vi "Remove Annotation.vi"(0 "FSM.Graph In":refnum<class "FSM.Graph.lvclass">, 7 "Name":string) -> (4 "FSM.Graph Out":refnum<class "FSM.Graph.lvclass">)   [LabVIEW 2020, in "FSM.Graph.lvclass"]
uses:
  FSM.Graph.lvclass
  FSM.Graph.lvclass/FSM.Graph.ctl
  FSM.Edge/FSM.Edge.lvclass
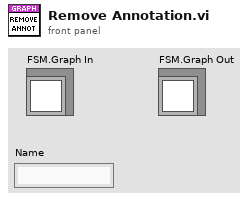
[diagram p1: front panel]
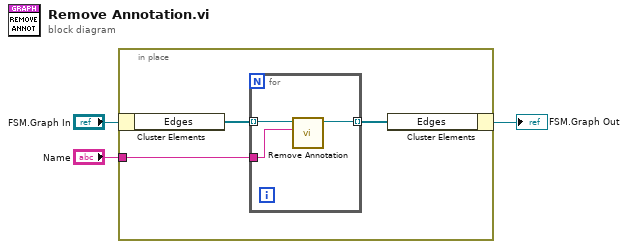
[diagram p0: block diagram]
diagram:
  n1 = in-place {
    in-place-border: "Name" -> [w5]
    n2 = in-place-cluster #1("FSM.Graph In") -> ("Edges"=w6:refnum<class "FSM.Edge.lvclass">[])
    n3 = for {
      tunnel: w6 -> [w9] mode=indexing
      tunnel: w5 -> [w8]
      tunnel: [w7] -> w4 mode=indexing
      n4 = call "Remove Annotation.vi"("Name"=w8, "FSM.Edge in"=w9) -> ("FSM.Edge out"=w7:refnum<class "FSM.Edge.lvclass">)  [unwired: 8 in, 1 out]
    }
    n5 = in-place-cluster #1("Edges"=w4) -> (→"FSM.Graph Out":refnum<class "FSM.Graph.lvclass">)
  }
